vi "LAUNCHER.vi"   [LabVIEW 2019]
uses:
  CAFE_MEX_ESP.lvclass
  C:/Program Files (x86)/National Instruments/LabVIEW 2019/vi.lib/ActorFramework/Actor/Actor.lvclass
  <vilib>/ActorFramework/Actor/Actor.lvclass
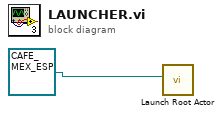
[diagram p0: block diagram]
diagram:
  n1 = call <vilib>:"Launch Root Actor.vi"("Actor"=refnum<class "CAFE_MEX_ESP.lvclass"> refnum ("CAFE_MEX_ESP.lvlib:CAFE_MEX_ESP.lvclass")) -> ()  [unwired: 9 in, 2 out]
